vi "DialogProgramError.vi"(7 "エラー内容":string, 10 "エラー詳細":string) -> (0 "error out":errorcluster caption="エラー出力")   [LabVIEW 2016]
panel:
  in  "btn":bool
  out "呼出履歴":string[](array[string])
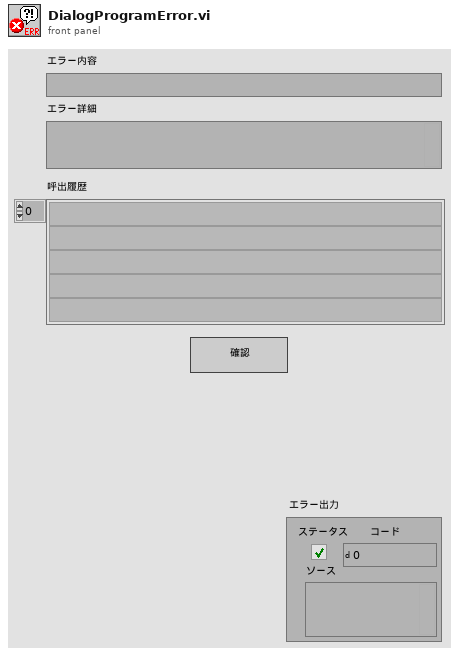
[diagram p1: front panel]
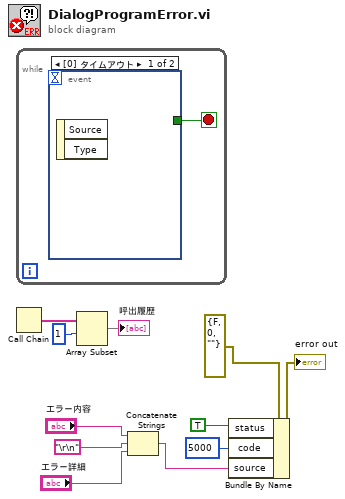
[diagram p0: block diagram]
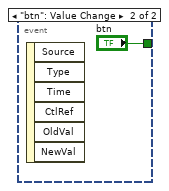
[diagram p2: hidden frame]
diagram:
  n1 = Call Chain() -> (call chain=w11:string[])
  n2 = while {
    stop <- w12 stop-if-true
    n3 = event shown="[0] タイムアウト" {
      selector: _ -> [_ _]
      dyn-events: _ -> [_ _]
      timeout: _ -> [_ _]
      tunnel: [_ "btn"] -> w12
      event Timeout {
        n4 = event-data() -> ()  [unwired: 1 in, 2 out]
      }
      event "btn": Value Change {
        n5 = event-data() -> ()  [unwired: 1 in, 6 out]
      }
    }
  }
  n6 = Array Subset(array=w11, index=1 ("指標")) -> (→"呼出履歴":string[])  [unwired: 1 in]
  n7 = Concatenate Strings("エラー内容", "\r\n", "エラー詳細") -> (w1:string)
  n8 = Bundle By Name(cluster=errorcluster {"status"=FALSE, "code"=0, "source"=""} ("エラー定数"), "status"=TRUE, "code"=5000, "source"=w1) -> (→"error out":errorcluster)
